vi "Response Handlers.vi"(4 "WebSocket Handler":refnum<class "WebSocket Handler.lvclass">, 9 "Response Handler Map":T1, 11 "Processing In":refnum<class "Processing.lvclass">) -> (0 "error out":errorcluster, 3 "HTTP Server.lvlib:Processing":refnum<class "Processing.lvclass">)   [LabVIEW 2020, in "HTTP Server.lvlib" / "Server.lvclass"]
uses:
  Server.lvclass
  Processing/Processing.lvclass
  Response Handler Map.ctl
  Priority.ctl
  Response Handler/Response Handler.lvclass
  WebSocket Handler/WebSocket Handler.lvclass
  C:/dev/lv20CE/relink/lv-http-server/HTTP Server/Handler/Handler.lvclass
  C:/dev/lv20CE/relink/lv-http-server/HTTP Server/Response Handler/Response Handler.lvclass
  Processing Step.ctl
  Processing/Processing.lvclass/Processing.ctl
  Handler/Handler.lvclass
  Server.lvclass/Server.ctl
  HTTP Server.lvlib
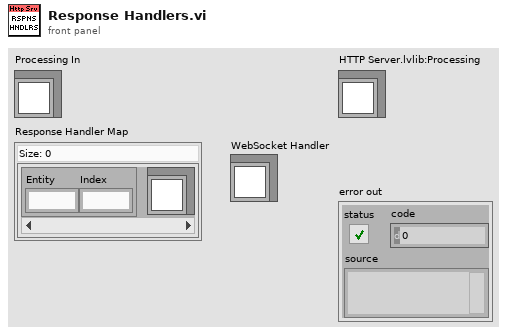
[diagram p1: front panel]
types:
  T1 = typedef "HTTP Server.lvlib/Response Handler Map.ctl" = map{T2, refnum<class "Response Handler.lvclass">}
  T2 = typedef "HTTP Server.lvlib/Priority.ctl" = cluster{"Entity":u16, "Index":u16}
  T3 = typedef "HTTP Server.lvlib/Processing Step.ctl" = enum16{"Connection", "Request", "Routing", "Controller Init", "Controller", "Response", "Complete", "Exception"}
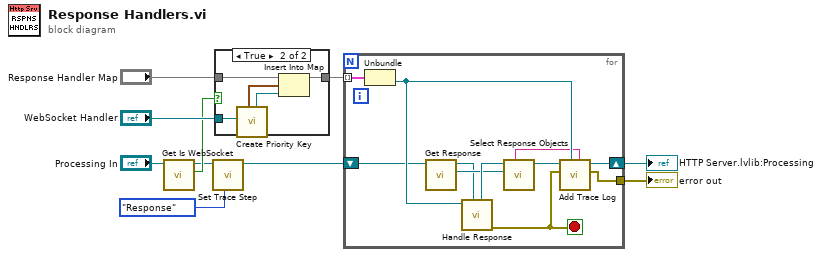
[diagram p0: block diagram]
diagram:
  n1 = call "Get Is WebSocket.vi"("Processing in"="Processing In") -> ("Is WebSocket"=w6:bool, "Processing out"=w5:refnum<class "Processing.lvclass">)  [unwired: 9 in]
  n2 = call "Set Trace Step.vi"("Processing Step"=Processing_Step."Response", "Processing in"=w5) -> ("Processing out"=w4:refnum<class "Processing.lvclass">)  [unwired: 9 in]
  n3 = case shown="True" w6 {
    tunnel: "Response Handler Map" -> [w11 w14]
    tunnel: "WebSocket Handler" -> [_ w12]
    tunnel: [w11 w13] -> w8
    frame False {
    }
    frame True {
      n4 = call "Create Priority Key.vi"("Handler In"=w12) -> ("Handler"=w15:refnum<class "WebSocket Handler.lvclass">, "Priority Key"=w16:T2)  [unwired: 8 in, 1 out]
      n5 = Insert Into Map(map in=w14, key=w16, value=w15) -> (map out=w13:T1)  [unwired: 2 out]
    }
  }
  n6 = for {
    tunnel: w8 -> [w27] mode=indexing
    shift-right: [w23] -> w3
    shift-left: w4 -> [w19]
    tunnel: [w20] -> w2
    stop <- w21 stop-if-true
    n7 = Unbundle(w27) -> ("Handler"=w25:refnum<class "Response Handler.lvclass">)  [unwired: 1 out]
    n8 = call "Get Response.vi"("Processing in"=w19) -> ("Response"=w18:refnum<class "Response.lvclass">, "Processing out"=w17:refnum<class "Processing.lvclass">)  [unwired: 9 in]
    n9 = call-dynamic "Handle Response.vi"("Processing In"=w17, "Response Handler in"=w25) -> ("error out"=w21:errorcluster, "Processing"=w22:refnum<class "Processing.lvclass">)  [unwired: 8 in]
    n10 = call "Select Response Objects.vi"("Response"=w18, "Response Inputs"=w22) -> ("Updated Inputs"=w26:refnum<class "Processing.lvclass">, "Trace Message"=w24:string)  [unwired: 8 in]
    n11 = call "Add Trace Log.vi"("Info"=w24, "LabVIEW Object"=w25, "error in (no error)"=w21, "Processing in"=w26) -> ("error out"=w20:errorcluster, "Processing out"=w23:refnum<class "Processing.lvclass">)  [unwired: 6 in]
  }
  "error out" <- w2
  "HTTP Server.lvlib:Processing" <- w3
